vi "Main.Read Data from VS.vi"(8 "error in":errorcluster, 11 "Data Sessions":T1[](array[typedef]) {"Outgoing.Frames.CountersAndProtections"."Protection Configurations"."CRC Channels"."Data Type" items=["Signed", "Unsigned", "IEEE Float"]; "Trigger.Refs"."Data Reference" format="%.0x"; "Disable.Refs"."Data Reference" format="%.0x"; "Timing.Refs"."Data Reference" format="%.0x"; "Network"."Name" format="%.0x"; "Incoming.Refs"."Data Reference" format="%.0x"; "Outgoing.Refs"."Data Reference" format="%.0x"}) -> (0 "error out":errorcluster, 3 "Data Sessions out":T1[](array[typedef]) {"Outgoing.Frames.CountersAndProtections"."Protection Configurations"."CRC Channels"."Data Type" items=["Signed", "Unsigned", "IEEE Float"]; "Trigger.Refs"."Data Reference" format="%.0x"; "Disable.Refs"."Data Reference" format="%.0x"; "Timing.Refs"."Data Reference" format="%.0x"; "Network"."Name" format="%.0x"; "Incoming.Refs"."Data Reference" format="%.0x"; "Outgoing.Refs"."Data Reference" format="%.0x"})   [LabVIEW 2019, in "J1939 Addon Engine.lvlib"]
uses:
  J1939 Addon Engine.lvlib
  Types/Protocol.XNET Refs.ctl
  Addon Shared/Types/Monitor Settings.ctl
  <vilib>/NI VeriStand/Custom Device API/Block Data Reference.ctl
  <vilib>/NI VeriStand/Custom Device API/Data Reference.ctl
  Types/Main.Outgoing.Frame.Settings.ctl
  Addon Shared/Types/Outgoing Event Trigger Types.ctl
  SubModules/Frame Protection Support/Source/Shared/Types/Exported Frame Settings.ctl
  SubModules/Frame Protection Support/Source/Shared/Types/Exported Frame Type.ctl
  SubModules/Frame Protection Support/Source/Shared/Types/Exported Protection Settings.ctl
  SubModules/Frame Protection Support/Source/Shared/Types/Protection Type.ctl
  SubModules/Frame Protection Support/Source/Shared/Types/XNET Signal Configuration.ctl
  SubModules/Frame Protection Support/Source/Shared/Types/Exported Counter Settings.ctl
  SubModules/Frame Protection Support/Source/Shared/Types/Exported Event Trigger Type.ctl
  <vilib>/xnet/xnet.llb/XNET Control Scope.ctl
  <vilib>/NI VeriStand/Custom Device API/Global Data Refs.vi
  <vilib>/xnet/xnet.llb/XNET Write (Signal Single-point).vi
  <vilib>/NI VeriStand/Custom Device API/Custom Device API.lvlib
  Addon Shared/J1939 Addon Shared.lvlib
  SubModules/Frame Protection Support/Source/Shared/Protection and Counter Support Shared.lvlib
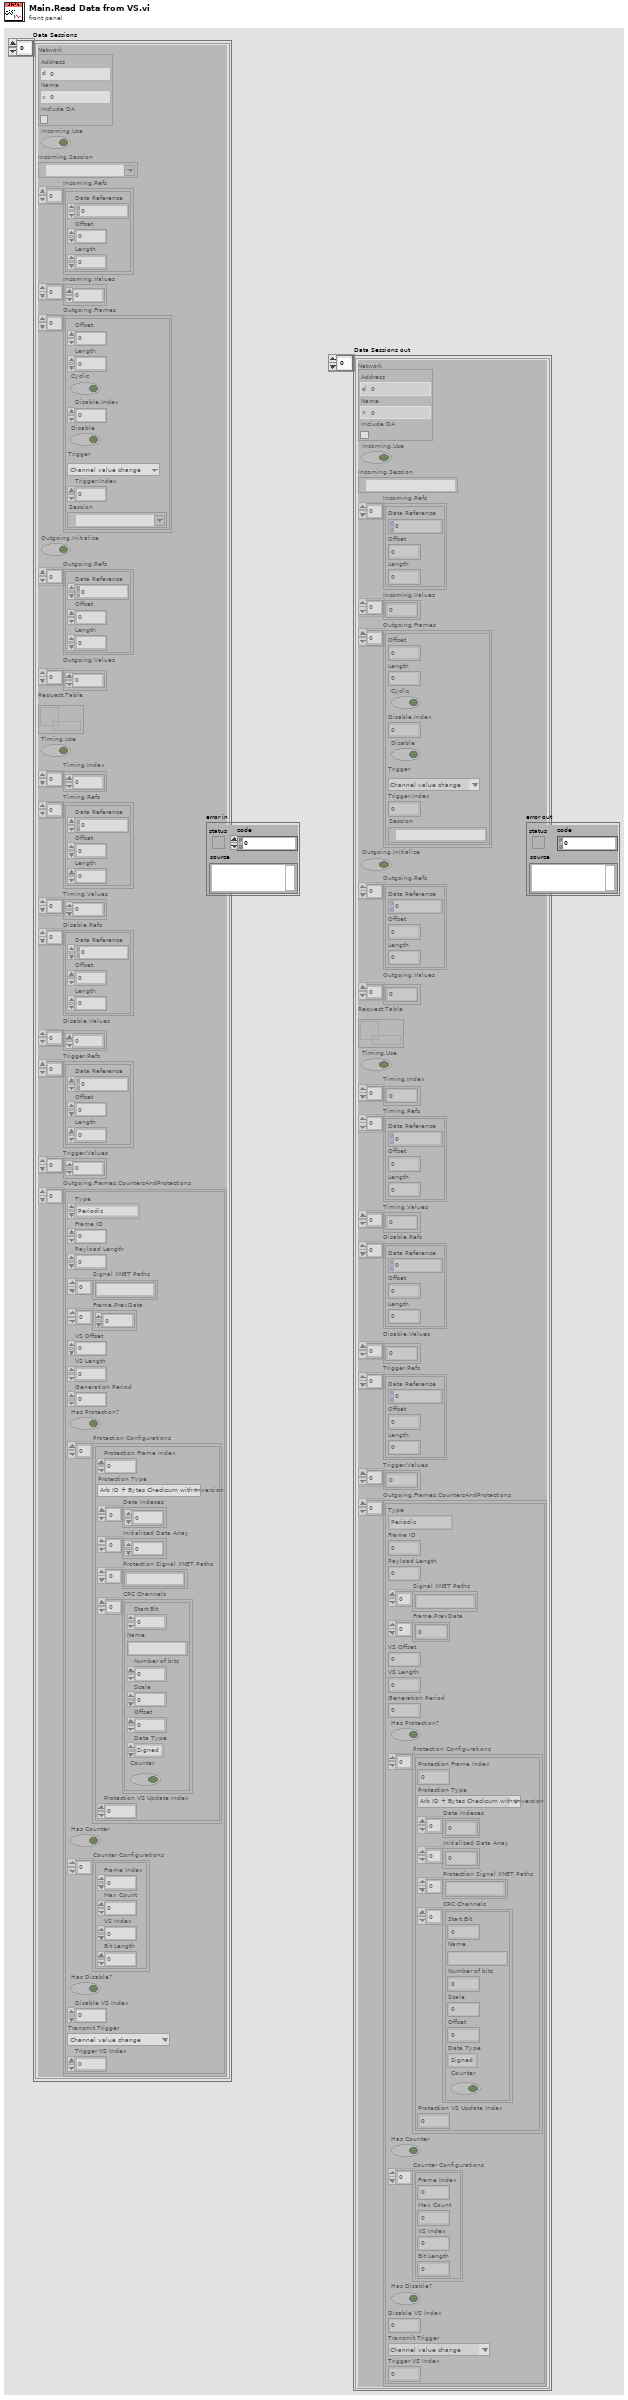
[diagram p1: front panel]
types:
  T1 = typedef "J1939 Addon Engine.lvlib/Protocol.XNET Refs.ctl" = cluster{"Network":T2, "Incoming.Use":bool, "Incoming.Session":refnum<k21>, "Incoming.Refs":T3[], "Incoming.Values":dbl[], "Outgoing.Frames":T5[], "Outgoing.Initialize":bool, "Outgoing.Refs":T3[], "Outgoing.Values":dbl[], "Request.Table":refnum<k33>, "Timing.Use":bool, "Timing.Index":i32[], "Timing.Refs":T3[], "Timing.Values":dbl[], "Disable.Refs":T3[], "Disable.Values":dbl[], "Trigger.Refs":T3[], "Trigger.Values":dbl[], "Outgoing.Frames.CountersAndProtections":T7[]}
  T2 = typedef "J1939 Addon Shared.lvlib/Monitor Settings.ctl" = cluster{"Address":u8, "Name":u64, "Include DA":bool}
  T3 = typedef "Custom Device API.lvlib/Block Data Reference.ctl" = cluster{"Data Reference":T4, "Offset":u64, "Length":u64}
  T4 = typedef "Custom Device API.lvlib/Data Reference.ctl" = i32
  T5 = typedef "J1939 Addon Engine.lvlib/Main.Outgoing.Frame.Settings.ctl" = cluster{"Offset":u32, "Length":u32, "Cyclic":bool, "Disable.Index":i32, "Disable":bool, "Trigger":T6, "Trigger.Index":i32, "Session":refnum<k21>}
  T6 = typedef "J1939 Addon Shared.lvlib/Outgoing Event Trigger Types.ctl" = enum16{"Channel value change", "Trigger channel (not zero)", "Channel value change or trigger channel (not zero)", "Trigger channel (any value change)", "Channel value change or trigger channel (any value change)"}
  T7 = typedef "Protection and Counter Support Shared.lvlib/Exported Frame Settings.ctl" = cluster{"Type":T8, "Frame ID":u32, "Payload Length":u32, "Signal XNET Paths":string[], "Frame.PrevData":dbl[], "VS Offset":i32, "VS Length":i32, "Generation Period":u32, "Has Protection?":bool, "Protection Configurations":T9[], "Has Counter":bool, "Counter Configurations":T12[], "Has Disable?":bool, "Disable VS Index":i32, "Transmit Trigger":T13, "Trigger VS Index":i32}
  T8 = typedef "Protection and Counter Support Shared.lvlib/Exported Frame Type.ctl" = enum16{"Periodic", "Event", "Periodic/Event"}
  T9 = typedef "Protection and Counter Support Shared.lvlib/Exported Protection Settings.ctl" = cluster{"Protection Frame Index":i32, "Protection Type":T10, "Data Indeces":i32[], "Initialized Data Array":dbl[], "Protection Signal XNET Paths":string[], "CRC Channels":T11[], "Protection VS Update Index":i32}
  T10 = typedef "Protection and Counter Support Shared.lvlib/Protection Type.ctl" = enum16{"Arb ID + Bytes Checksum with Inversion", "Arb ID + Bytes CRC with Inversion", "Reversed Raw Signal Checksum with Inversion", "Concatenated Two's Compliment"}
  T11 = typedef "Protection and Counter Support Shared.lvlib/XNET Signal Configuration.ctl" = cluster{"Start Bit":i32, "Name":string, "Number of bits":i32, "Scale":dbl, "Offset":dbl, "Data Type":u32, "Counter":bool}
  T12 = typedef "Protection and Counter Support Shared.lvlib/Exported Counter Settings.ctl" = cluster{"Frame Index":i32, "Max Count":dbl, "VS Index":i32, "Bit Length":i64}
  T13 = typedef "Protection and Counter Support Shared.lvlib/Exported Event Trigger Type.ctl" = enum16{"Channel value change", "Trigger channel (not zero)", "Channel value change or trigger channel (not zero)", "Trigger channel (any value change)", "Channel value change or trigger channel (any value change)"}
  T14 = typedef "XNET Control Scope.ctl" = u32
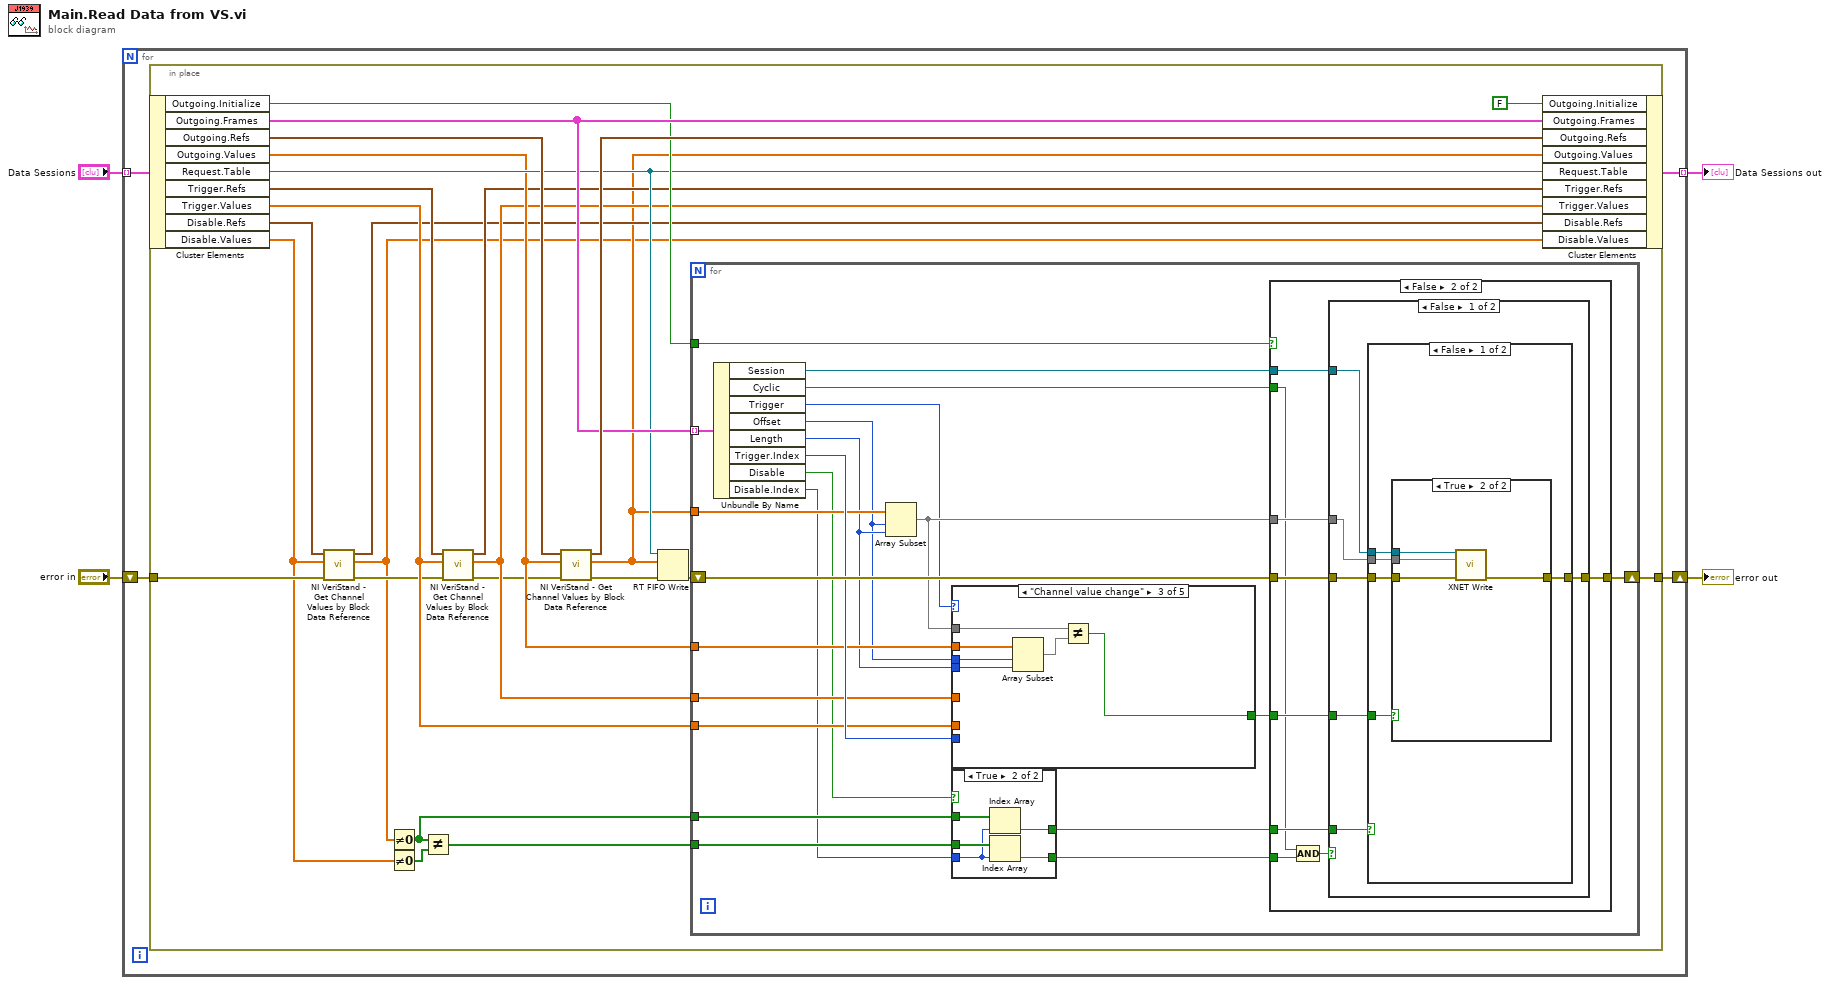
[diagram p0: block diagram]
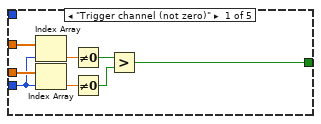
[diagram p2: hidden frame]
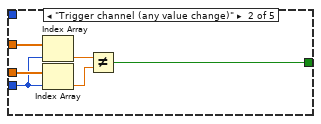
[diagram p3: hidden frame]
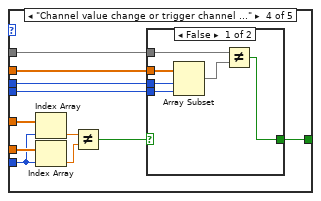
[diagram p4: hidden frame]
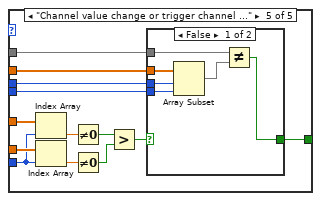
[diagram p6: hidden frame]
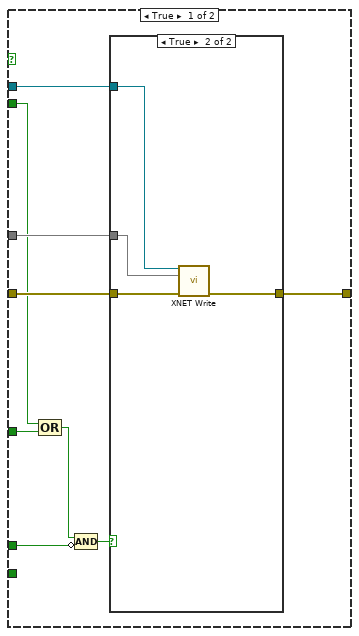
[diagram p9: hidden frame]
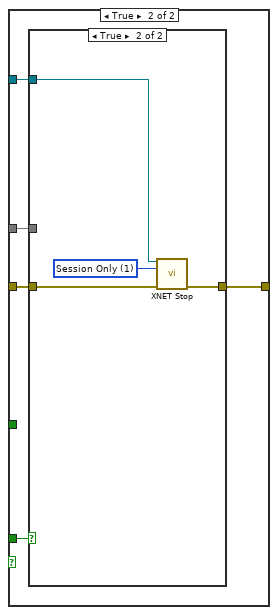
[diagram p13: hidden frame]
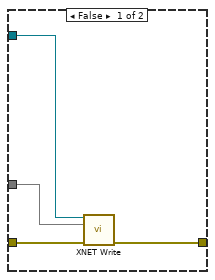
[diagram p14: hidden frame]
diagram:
  n1 = for {
    shift-right: [w7] -> w1
    shift-left: "error in" -> [w8]
    tunnel: "Data Sessions" -> [w6] mode=indexing
    tunnel: [w5] -> w3 mode=indexing
    n2 = in-place {
      in-place-border: w8 -> [w16]
      in-place-border: [w26] -> w7
      n3 = in-place-cluster #1(w6) -> ("Outgoing.Initialize"=w29:bool, "Outgoing.Frames"=w31:T5[], "Outgoing.Refs"=w33:T3[], "Outgoing.Values"=w24:dbl[], "Request.Table"=w25:refnum<k33>, "Trigger.Refs"=w22:T3[], "Trigger.Values"=w19:dbl[], "Disable.Refs"=w15:T3[], "Disable.Values"=w10:dbl[])
      n4 = call <vilib>:"NI VeriStand - Get Channel Values by Block Data Reference.vi"("error in (no error)"=w16, "Values Array in"=w10, "Block Data Ref"=w15) -> ("error out"=w17:errorcluster, "Values Array out"=w11:dbl[], "Block Data Ref dup"=w14:T3[])  [unwired: 6 in]
      n5 = Not Equal To 0?(x=w11) -> (x != 0?=w23:bool[])
      n6 = Not Equal To 0?(x=w10) -> (x != 0?=w9:bool[])
      n7 = Not Equal?(x=w23, y=w9) -> (x != y?=w13:bool[])
      n8 = call <vilib>:"NI VeriStand - Get Channel Values by Block Data Reference.vi"("error in (no error)"=w17, "Values Array in"=w19, "Block Data Ref"=w22) -> ("error out"=w18:errorcluster, "Values Array out"=w20:dbl[], "Block Data Ref dup"=w21:T3[])  [unwired: 6 in]
      n9 = call <vilib>:"NI VeriStand - Get Channel Values by Block Data Reference.vi"("error in (no error)"=w18, "Values Array in"=w24, "Block Data Ref"=w33) -> ("error out"=w28:errorcluster, "Values Array out"=w12:dbl[], "Block Data Ref dup"=w32:T3[])  [unwired: 6 in]
      n10 = RT FIFO Write(0:w25, 1:w12, 3:w28) -> (11:w27:errorcluster)  [unwired: 2 in, 3 out]
      n11 = for {
        tunnel: w12 -> [w42]
        tunnel: w31 -> [w53] mode=indexing
        tunnel: w24 -> [w40]
        shift-right: [w55] -> w26
        shift-left: w27 -> [w54]
        tunnel: w29 -> [w52]
        tunnel: w13 -> [w50]
        tunnel: w23 -> [w48]
        tunnel: w20 -> [w45]
        tunnel: w19 -> [w44]
        n12 = Unbundle By Name(w53) -> ("Session"=w34:refnum<k21>, "Cyclic"=w51:bool, "Trigger"=w36:T6, "Offset"=w38:u32, "Length"=w39:u32, "Trigger.Index"=w46:i32, "Disable"=w37:bool, "Disable.Index"=w35:i32)
        n13 = Array Subset(array=w42, index=w38, length=w39) -> (w41:dbl[])
        n14 = case shown="\"Channel value change\"" w36 {
          tunnel: w46 -> [w59 w65 _ w78 w95]
          tunnel: w45 -> [w61 w67 _ w80 w97]
          tunnel: w44 -> [w60 w66 _ w79 w96]
          tunnel: [w56 w64 w74 w86 w106] -> w43
          tunnel: w40 -> [_ _ w73 w85 w105]
          tunnel: w41 -> [_ _ w72 w84 w104]
          tunnel: w39 -> [_ _ w71 w83 w103]
          tunnel: w38 -> [_ _ w70 w82 w102]
          frame "Trigger channel (not zero)" {
            n15 = Index Array(array=w61, index=w59) -> (element=w62:dbl)
            n16 = Index Array(array=w60, index=w59) -> (element=w63:dbl)
            n17 = Not Equal To 0?(x=w62) -> (x != 0?=w57:bool)
            n18 = Not Equal To 0?(x=w63) -> (x != 0?=w58:bool)
            n19 = Greater?(x=w57, y=w58) -> (0:w56:bool)
          }
          frame "Trigger channel (any value change)" {
            n20 = Index Array(array=w67, index=w65) -> (element=w68:dbl)
            n21 = Index Array(array=w66, index=w65) -> (element=w69:dbl)
            n22 = Not Equal?(x=w68, y=w69) -> (x != y?=w64:bool)
          }
          frame "Channel value change" {
            n23 = Array Subset(array=w73, index=w70, length=w71) -> (w75:dbl[])
            n24 = Not Equal?(x=w72, y=w75) -> (x != y?=w74:bool)
          }
          frame "Channel value change or trigger channel (not zero)" {
            n25 = Index Array(array=w80, index=w78) -> (element=w81:dbl)
            n26 = Index Array(array=w79, index=w78) -> (element=w77:dbl)
            n27 = Not Equal?(x=w81, y=w77) -> (x != y?=w76:bool)
            n28 = case shown="False" w76 {
              selector: w76 -> [_ w93]
              tunnel: [w91 w93] -> w86
              tunnel: w85 -> [w90 _]
              tunnel: w84 -> [w89 _]
              tunnel: w83 -> [w88 _]
              tunnel: w82 -> [w87 _]
              frame False {
                n29 = Array Subset(array=w90, index=w87, length=w88) -> (w92:dbl[])
                n30 = Not Equal?(x=w89, y=w92) -> (x != y?=w91:bool)
              }
              frame True {
              }
            }
          }
          frame "Channel value change or trigger channel (any value change)" {
            n31 = Index Array(array=w97, index=w95) -> (element=w100:dbl)
            n32 = Index Array(array=w96, index=w95) -> (element=w101:dbl)
            n33 = Not Equal To 0?(x=w100) -> (x != 0?=w98:bool)
            n34 = Not Equal To 0?(x=w101) -> (x != 0?=w99:bool)
            n35 = Greater?(x=w98, y=w99) -> (0:w94:bool)
            n36 = case shown="False" w94 {
              selector: w94 -> [_ w113]
              tunnel: [w111 w113] -> w106
              tunnel: w105 -> [w110 _]
              tunnel: w104 -> [w109 _]
              tunnel: w103 -> [w108 _]
              tunnel: w102 -> [w107 _]
              frame False {
                n37 = Array Subset(array=w110, index=w107, length=w108) -> (w112:dbl[])
                n38 = Not Equal?(x=w109, y=w112) -> (x != y?=w111:bool)
              }
              frame True {
              }
            }
          }
        }
        n39 = case shown="True" w37 {
          selector: w37 -> [w114 _]
          tunnel: w50 -> [_ w119]
          tunnel: w35 -> [_ w117]
          tunnel: [w114 w116] -> w49
          tunnel: w48 -> [_ w118]
          tunnel: [w114 w115] -> w47
          frame False {
          }
          frame True {
            n40 = Index Array(array=w118, index=w117) -> (element=w116:bool)
            n41 = Index Array(array=w119, index=w117) -> (element=w115:bool)
          }
        }
        n42 = case shown="False" w52 {
          tunnel: [w128 w142] -> w55
          tunnel: w54 -> [w127 w141]
          tunnel: w34 -> [w126 w140]
          tunnel: w41 -> [w125 w139]
          tunnel: w51 -> [w122 w134]
          tunnel: w43 -> [w121 w138]
          tunnel: w49 -> [w123 w137]
          tunnel: w47 -> [_ w136]
          frame True {
            n43 = Compound Arithmetic op=OR(w122, w121) -> (w120:bool)
            n44 = Compound Arithmetic op=AND(w120, invert w123) -> (w124:bool)
            n45 = case shown="True" w124 {
              tunnel: [w129 w130] -> w128
              tunnel: w127 -> [w129 w132]
              tunnel: w126 -> [_ w131]
              tunnel: w125 -> [_ w133]
              frame False {
              }
              frame True {
                n46 = call-poly <vilib>:"XNET Write.vi"("session in"=w131, "data"=w133, "error in (no error)"=w132) -> ("error out"=w130:errorcluster)  [unwired: 11 in, 1 out]
              }
            }
          }
          frame False {
            n47 = Compound Arithmetic op=AND(w134, w136) -> (w135:bool)
            n48 = case shown="False" w135 {
              tunnel: [w148 w161] -> w142
              tunnel: w141 -> [w147 w162]
              tunnel: w140 -> [w146 w163]
              tunnel: w139 -> [w145 w160]
              tunnel: w138 -> [w144 _]
              tunnel: w137 -> [w143 w164]
              frame False {
                n49 = case shown="False" w143 {
                  tunnel: [w153 w159] -> w148
                  tunnel: w147 -> [w152 w159]
                  tunnel: w146 -> [w151 _]
                  tunnel: w145 -> [w150 _]
                  tunnel: w144 -> [w149 _]
                  frame False {
                    n50 = case shown="True" w149 {
                      tunnel: [w154 w158] -> w153
                      tunnel: w152 -> [w154 w157]
                      tunnel: w151 -> [_ w156]
                      tunnel: w150 -> [_ w155]
                      frame False {
                      }
                      frame True {
                        n51 = call-poly <vilib>:"XNET Write.vi"("session in"=w156, "data"=w155, "error in (no error)"=w157) -> ("error out"=w158:errorcluster)  [unwired: 11 in, 1 out]
                      }
                    }
                  }
                  frame True {
                  }
                }
              }
              frame True {
                n52 = case shown="True" w164 {
                  tunnel: w163 -> [w166 w172]
                  tunnel: w162 -> [w167 w171]
                  tunnel: [w165 w170] -> w161
                  tunnel: w160 -> [w168 _]
                  frame False {
                    n53 = call-poly <vilib>:"XNET Write.vi"("session in"=w166, "data"=w168, "error in (no error)"=w167) -> ("error out"=w165:errorcluster)  [unwired: 11 in, 1 out]
                  }
                  frame True {
                    w169 = T14 1 items=["Normal", "Session Only", "Interface Only", "Session Only Blocking"] ("scope (normal)")
                    n54 = call <vilib>:"XNET Stop.vi"("session in"=w172, "scope (normal)"=w169, "error in (no error)"=w171) -> ("error out"=w170:errorcluster)  [unwired: 11 in, 1 out]
                  }
                }
              }
            }
          }
        }
      }
      n55 = in-place-cluster #1("Outgoing.Initialize"=FALSE ("Initialize Outgoing?"), "Outgoing.Frames"=w31, "Outgoing.Refs"=w32, "Outgoing.Values"=w12, "Request.Table"=w25, "Trigger.Refs"=w21, "Trigger.Values"=w20, "Disable.Refs"=w14, "Disable.Values"=w11) -> (w5:T1)
    }
  }
  "Data Sessions out" <- w3
  "error out" <- w1
